vi "mean_values_2Darray.vi"(6 "error in (no error)":errorcluster, 9 "Array":dbl[][](array[numeric])) -> (0 "error out":errorcluster, 3 "mean values":dbl[](array[numeric]))   [LabVIEW 2010]
uses:
  <vilib>/Analysis/NI_AALBase.lvlib
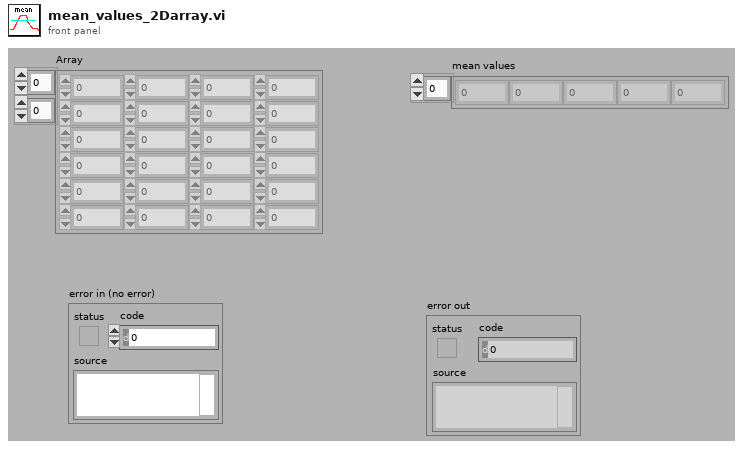
[diagram p1: front panel]
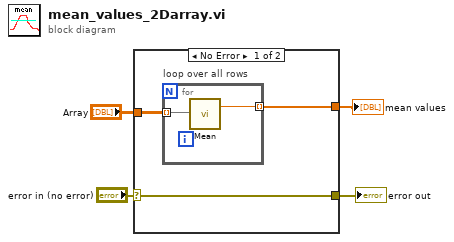
[diagram p0: block diagram]
diagram:
  n1 = case shown="No Error" "error in (no error)" {
    selector: "error in (no error)" -> [w6 w10]
    tunnel: "Array" -> [w7 _]
    tunnel: [w5 _] -> w3
    tunnel: [w6 w10] -> w1
    frame No Error {
      n2 = for "loop over all rows" {
        tunnel: w7 -> [w9] mode=indexing
        tunnel: [w8] -> w5 mode=indexing
        n3 = call <vilib>:"Mean.vi"("X"=w9) -> ("mean"=w8:dbl)  [unwired: 1 out]
      }
    }
    frame Error {
    }
  }
  "mean values" <- w3
  "error out" <- w1
